vi "SendPacket.vi"(8 "error in (no error)":errorcluster, 9 "EscapePattern":T1, 10 "Transmit":T2, 11 "VISA resource name":refnum<visa-resource-name>) -> (0 "error out":errorcluster, 3 "VISA resource name out":refnum<visa-resource-name>)   [LabVIEW 2009]
uses:
  Packet.ctl
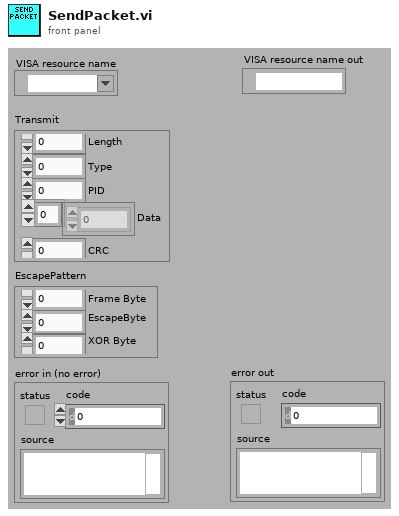
[diagram p1: front panel]
types:
  T1 = cluster{"Frame Byte":u8, "EscapeByte":u8, "XOR Byte":u8}
  T2 = typedef "Packet.ctl" = cluster{"Length":u8, "Type":u8, "PID":u8, "Data":u8[], "CRC":u8}
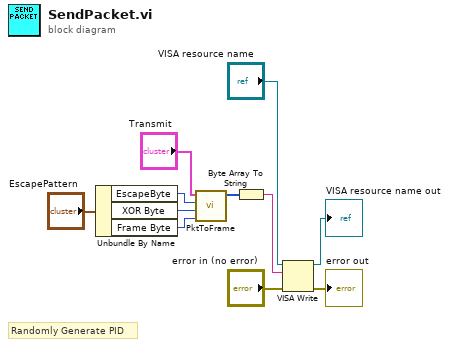
[diagram p0: block diagram]
diagram:
  # "Randomly Generate PID"
  n1 = Unbundle By Name("EscapePattern") -> ("EscapeByte"=w7:u8, "XOR Byte"=w6:u8, "Frame Byte"=w5:u8)
  n2 = call "PktToFrame.vi"("FrameByte"=w5, "XORByte"=w6, "EscapeByte"=w7, "Packet"="Transmit") -> ("Data"=w11:u8[])  [unwired: 7 in]
  n3 = Byte Array To String(unsigned byte array=w11) -> (string=w10:string)
  n4 = VISA Write(VISA resource name="VISA resource name", write buffer=w10, error in (no error)="error in (no error)") -> (VISA resource name out=→"VISA resource name out":refnum<visa-resource-name>, error out=→"error out":errorcluster)  [unwired: 1 out]
